vi "Digital Output - 1 Channel - N Samples.vi"() -> ()   [LabVIEW 2019]
uses:
  <vilib>/myRIO/Common/Instrument Driver Framework/ELVIS III v1.0/DO Block/vis/ELVIS III v1.0 DO Block Write.vi
  <vilib>/myRIO/Common/Instrument Driver Framework/ELVIS III v1.0/DO Block/vis/ELVIS III v1.0 Close DO Block.vi
  <vilib>/myRIO/Common/Instrument Driver Framework/myRIO v1.0/UART/vis/myRIO v1.0 Close UART.vi
  <vilib>/myRIO/Common/Instrument Driver Framework/Utilities/vis/Sample Rate To Ticks.vi
  <vilib>/myRIO/Common/Instrument Driver Framework/ELVIS III v1.0/DO Block/vis/ELVIS III v1.0 Unreserve DO Block.vi
  <vilib>/myRIO/Common/Instrument Driver Framework/ELVIS III v1.0/DO Block/vis/ELVIS III v1.0 Build MUX Configuration DO Block.vi
  <vilib>/myRIO/Common/Instrument Driver Framework/ELVIS III v1.0/Resource Manager/vis/ELVIS III v1.0 Create Configuration List.vi
  <vilib>/Waveform/DWDTOps.llb/Digital Pattern Generator (Ramp).vi
  <vilib>/Waveform/DWDTOps.llb/DWDT Digital to Boolean Array.vi
  <vilib>/Utility/error.llb/Error Cluster From Error Code.vi
  <vilib>/myRIO/Common/Instrument Driver Framework/myRIO v1.0/Resource Manager/vis/myRIO v1.0 Block Write Configuration.vi
  <vilib>/myRIO/Common/Instrument Driver Framework/ELVIS III v1.0/DO Block/vis/ELVIS III v1.0 DO Build Bank Data.vi
  <vilib>/myRIO/Common/Instrument Driver Framework/ELVIS III v1.0/DO Block/vis/ELVIS III v1.0 DO Enqueue Data.vi
  <vilib>/myRIO/Common/Instrument Driver Framework/ELVIS III v1.0/Resource Manager/vis/ELVIS III v1.0 Configure IO.vi
  <vilib>/myRIO/Common/Instrument Driver Framework/ELVIS III v1.0/Resource Manager/vis/ELVIS III v1.0 Configure DO DIR.vi
  <vilib>/myRIO/Common/Instrument Driver Framework/ELVIS III v1.0/Resource Manager/vis/ELVIS III v1.0 Unreserve Channel List.vi
  <vilib>/myRIO/Common/Instrument Driver Framework/myRIO v1.0/myRIO v1.0 Close.vi
  <vilib>/myRIO/Common/Instrument Driver Framework/Utilities/vis/FPGA Ref Manager.vi
  <vilib>/myRIO/Common/Instrument Driver Framework/ELVIS III v1.0/ELVIS III v1.0 Reset FPGA.vi
  <vilib>/myRIO/Common/Instrument Driver Framework/myRIO v1.0/IRQ/vis/myRIO v1.0 IRQ Info FGV.vi
  <vilib>/myRIO/Common/Instrument Driver Framework/myRIO v1.0/IRQ/vis/myRIO v1.0 Timer IRQ Info FGV.vi
  <vilib>/myRIO/Common/Instrument Driver Framework/myRIO v1.0/IRQ/vis/myRIO v1.0 ISR Agent.vi
  <vilib>/myRIO/Instrument Drivers/Utilities/vis/Reset Index.vi
  <vilib>/myRIO/Common/Instrument Driver Framework/myRIO v1.0/Resource Manager/vis/myRIO v1.0 Block Write Resource Manager.vi
  <vilib>/myRIO/Instrument Drivers/Utilities/Utilities.lvlib
  <vilib>/myRIO/Instrument Drivers/Onboard IO/DO Block/DO Block.lvlib
panel:
  in  "Generate Ramp":bool
  out "Digital Waveform Graph":digitalwaveform(graph)
  in  "Stop":bool
  # "ELVIS III Control IO"
  # "数字输出单通道"
  # "Overview: Generates N sample digital output on Bank A, Channel DIO0 (A/DIO0).\nInstructions:\n1. Connect channel A/DIO0 to the positive lead of the load, and connect DGND to the negative lead of the load. DGND is the ground reference terminal for digital channels.\n2. Run the VI.\n3. Click Generate Ramp to trigger the digital output."
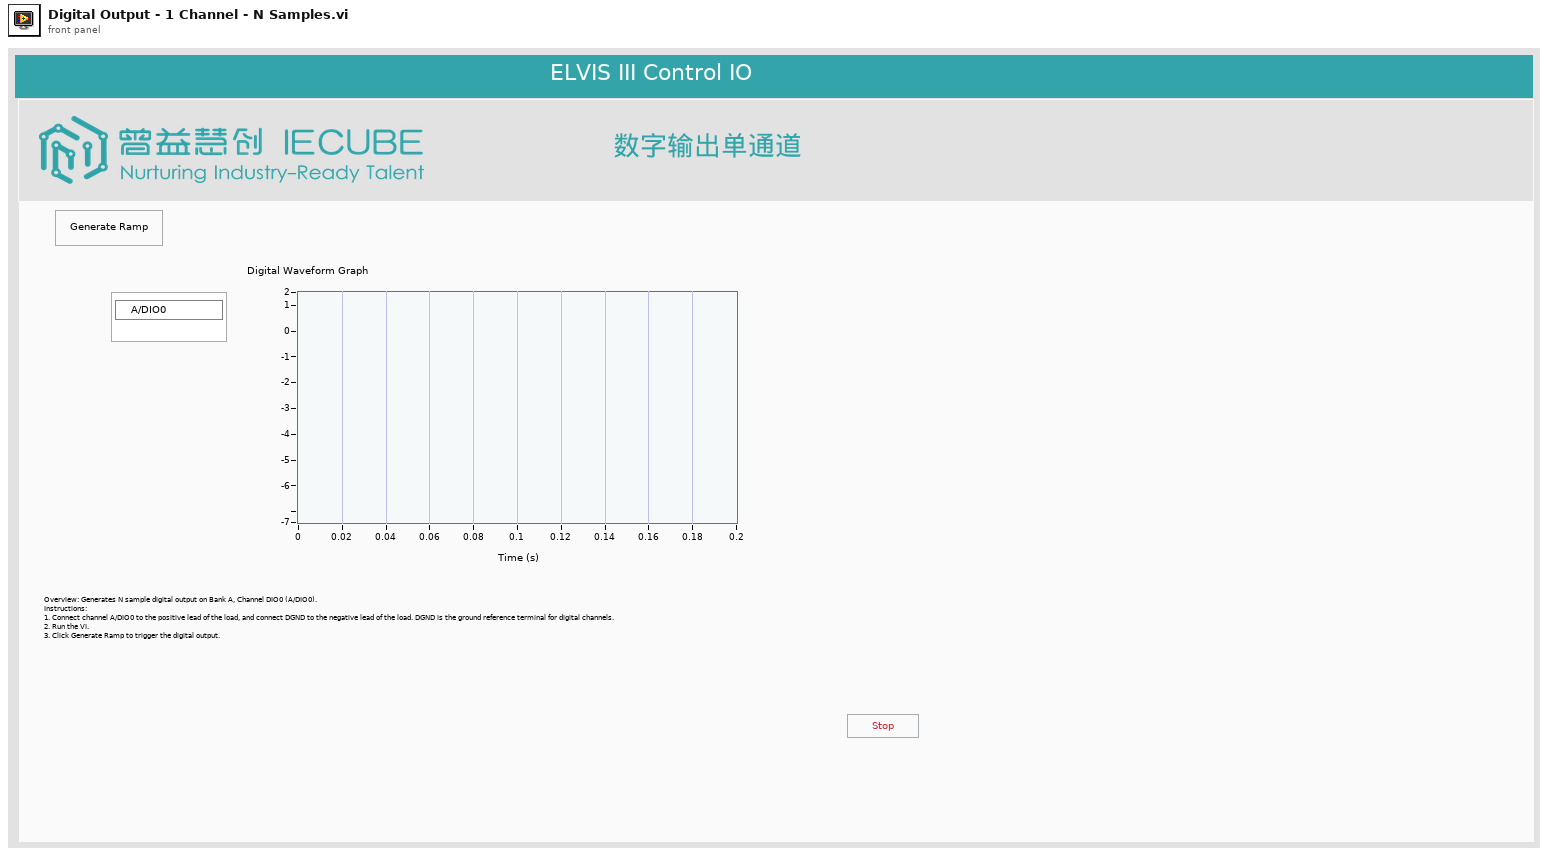
[diagram p1: front panel]
types:
  T1 = typedef "DO Block.lvlib/DO Block Reference.ctl" = cluster{"myRIO Reference":T2, "DO (N Samples) Channels List":T6}
  T2 = typedef "myRIO Generic Hardware Reference.ctl" = cluster{"myRIO Model":T3, "myRIO Hardware Reference":T4}
  T3 = typedef "Hardware Version Enum.ctl" = enum16{"Unknown", "myRIO-1900", "myRIO-1950", "roboRIO", "NI ELVIS RIO CM", "ELVIS III"}
  T4 = typedef "myRIO v1.0 Reference.ctl" = cluster{"Generic FPGA Reference":T5, "Allow multiple opens":bool}
  T5 = typedef "Generic FPGA Reference.ctl" = refnum<k20>
  T6 = typedef "DO Block Channels List.ctl" = T7[]
  T7 = typedef "DO Block Channels Enum.ctl" = enum16{"Not Connected", "A/DO0 (N Samples)", "A/DO1 (N Samples)", "A/DO2 (N Samples)", "A/DO3 (N Samples)", "A/DO4 (N Samples)", "A/DO5 (N Samples)", "A/DO6 (N Samples)", "A/DO7 (N Samples)", "A/DO8 (N Samples)", "A/DO9 (N Samples)", "A/DO10 (N Samples)", "A/DO11 (N Samples)", "A/DO12 (N Samples)", "A/DO13 (N Samples)", "A/DO14 (N Samples)", "A/DO15 (N Samples)", "A/DO16 (N Samples)", "A/DO17 (N Samples)", "A/DO18 (N Samples)", "A/DO19 (N Samples)", "B/DO0 (N Samples)", "B/DO1 (N Samples)", "B/DO2 (N Samples)", "B/DO3 (N Samples)", "B/DO4 (N Samples)", "B/DO5 (N Samples)", "B/DO6 (N Samples)", "B/DO7 (N Samples)", "B/DO8 (N Samples)", "B/DO9 (N Samples)", "B/DO10 (N Samples)", "B/DO11 (N Samples)", "B/DO12 (N Samples)", "B/DO13 (N Samples)", "B/DO14 (N Samples)", "B/DO15 (N Samples)", "B/DO16 (N Samples)", "B/DO17 (N Samples)", "B/DO18 (N Samples)", "B/DO19 (N Samples)"}
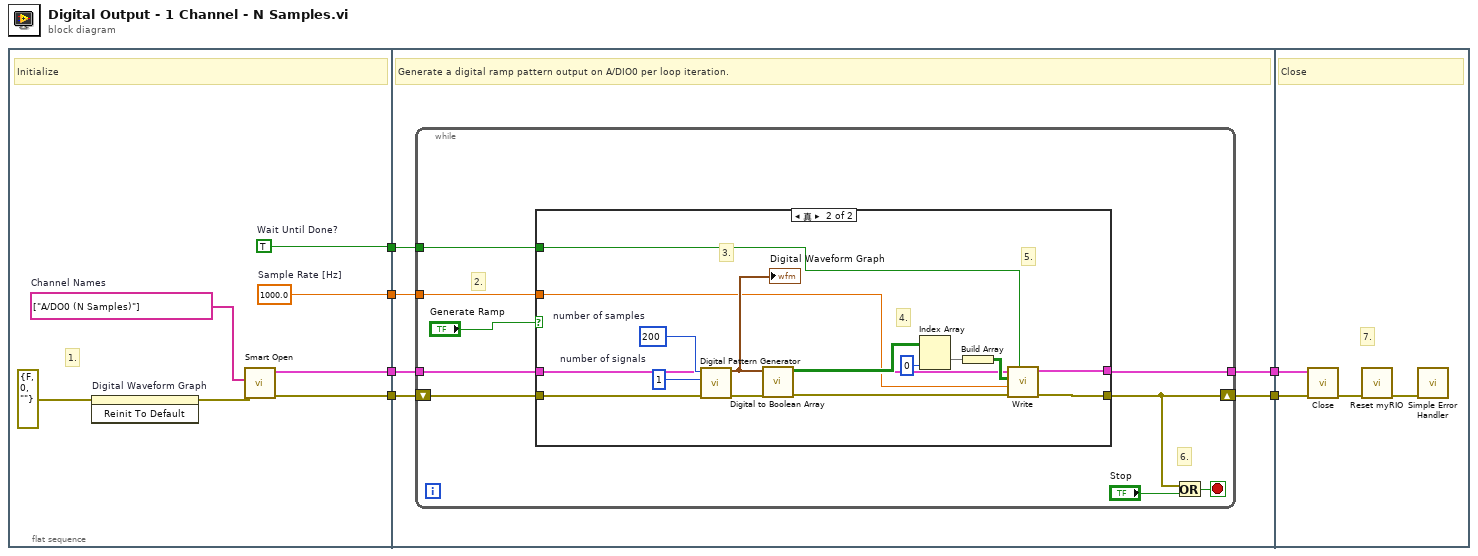
[diagram p0: block diagram]
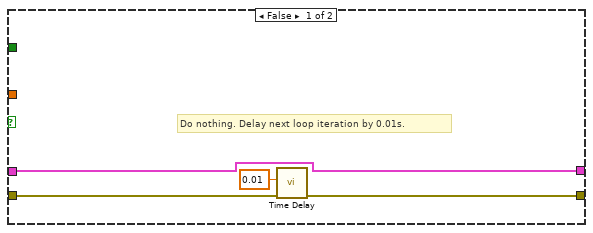
[diagram p2: hidden frame]
diagram:
  n1 = flat-sequence {
    tunnel: [w10] -> w6
    tunnel: [w9] -> w4
    tunnel: [w8] -> w3
    tunnel: [w7] -> w2
    tunnel: [w19] -> w5
    tunnel: w6 -> [w18]
    tunnel: w4 -> [w17]
    tunnel: w3 -> [w15]
    tunnel: w2 -> [w16]
    tunnel: [w14] -> w1
    tunnel: w5 -> [w50]
    tunnel: w1 -> [w48]
    frame #0 {
      w8 = TRUE  # Wait Until Done?
      w7 = 1000.0  # Sample Rate [Hz]
      w12 = tag[] ["A/DO0 (N Samples)"]  # Channel Names
      # "1."
      # "Initialize"
      n2 = invoke on="Digital Waveform Graph" class="DigitalGraph (strict)" method="Reinit To Default"(error in=errorcluster {"status"=FALSE, "code"=0, "source"=""} ("Error In")) -> (error out=w11:errorcluster)  [unwired: 2 in, 2 out]
      n3 = call <vilib>:"Smart Open.vi"("error in (no error)"=w11, "Channel Names"=w12) -> ("error out"=w10:errorcluster, "DO (N Samples) Ref Out"=w9:T1)  [unwired: 8 in]
    }
    frame #1 {
      # "Generate a digital ramp pattern output on A/DIO0 per loop iteration."
      n4 = while {
        shift-right: [w26] -> w19
        shift-left: w18 -> [w25]
        tunnel: w17 -> [w23]
        tunnel: w16 -> [w22]
        tunnel: w15 -> [w21]
        tunnel: [w20] -> w14
        stop <- w28 stop-if-true
        # "6."
        # "2."
        n5 = case shown="真" "Generate Ramp" {
          tunnel: [w31 w39] -> w26
          tunnel: w25 -> [w30 w42]
          tunnel: w23 -> [w29 w36]
          tunnel: [w29 w35] -> w20
          tunnel: w22 -> [_ w34]
          tunnel: w21 -> [_ w33]
          frame False {
            # "Do nothing. Delay next loop iteration by 0.01s."
            n6 = call "Time Delay"("error in (no error)"=w30, "Delay Time (s)"=0.01) -> ("error out"=w31:errorcluster)  [unwired: 9 in]
          }
          frame True {
            w44 = u32 200  # number of samples
            w43 = u32 1  # number of signals
            # "5."
            # "4."
            # "3."
            n7 = call-poly <vilib>:"Digital Pattern Generator.vi"("error in (no error)"=w42, "number of signals"=w43, "number of samples"=w44) -> ("error out"=w47:errorcluster, "digital waveform"=w41:digitalwaveform)  [unwired: 7 in]
            "Digital Waveform Graph" <- w41
            n8 = call-poly <vilib>:"Digital to Boolean Array.vi"("error in (no error)"=w47, "digital waveform"=w41) -> ("error out"=w40:errorcluster, "boolean array"=w45:bool[][])  [unwired: 8 in]
            n9 = Index Array(array=w45, index (col)=0 ("disabled index (col)")) -> (element=w38:bool[])  [unwired: 1 in]
            n10 = Build Array(w38) -> (w37:bool[][])
            n11 = call <vilib>:"Write.vi"("Wait Until Done?"=w33, "error in (no error)"=w40, "Sample Rate [Hz]"=w34, "Values"=w37, "DO (N Samples) Ref In"=w36) -> ("error out"=w39:errorcluster, "DO (N Samples) Ref Out"=w35:T1)  [unwired: 5 in]
          }
        }
        n12 = Or(x=w26, y="Stop") -> (x .or. y?=w28:bool)
      }
    }
    frame #2 {
      # "7."
      # "Close"
      n13 = call <vilib>:"Close.vi"("error in (no error)"=w50, "DO (N Samples) Ref In"=w48) -> ("error out"=w49:errorcluster)  [unwired: 9 in]
      n14 = call <vilib>:"Reset myRIO.vi"("error in (no error)"=w49) -> ("error out"=w51:errorcluster)  [unwired: 10 in]
      n15 = call <vilib>:"Simple Error Handler.vi"("error in (no error)"=w51) -> ()  [unwired: 4 in, 5 out]
    }
  }
